vi "Upload File.vi"(7 "Remote Folder Path":string, 8 "error in (no error)":errorcluster, 9 "Connection Name":string, 10 "Local File Path":path, 11 "Remote File Name":string) -> (0 "error out":errorcluster, 3 "Return String":string)   [LabVIEW 2019, in "LabSFTP.lvlib"]
doc: "<License>This software is distributed under the BSD 3-Clause License. For the full license please see license.txt or visit www.labvolution.com/license</License>"
uses:
  LabSFTP.lvlib
  FGV State..enum.ctl
  References/LabSFTP.dll
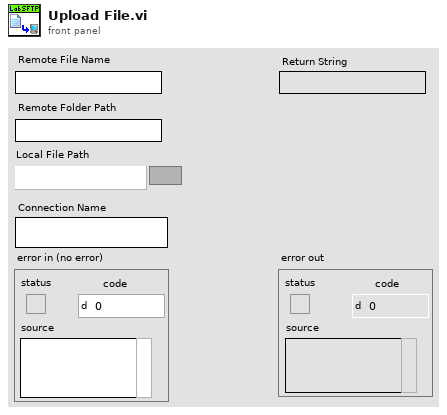
[diagram p1: front panel]
types:
  T1 = typedef "LabSFTP.lvlib/FGV State..enum.ctl" = enum16{"GET", "SET"}
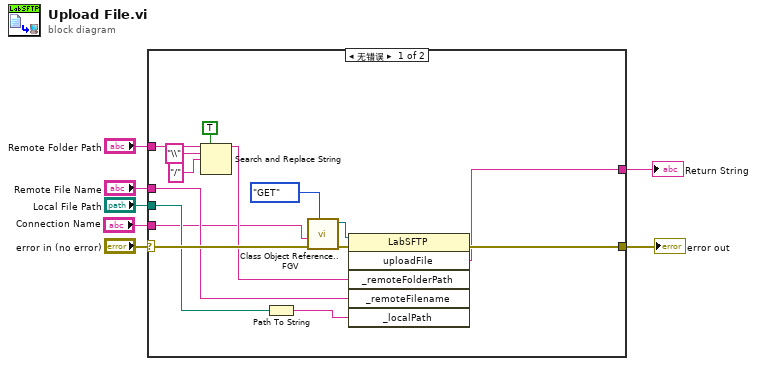
[diagram p0: block diagram]
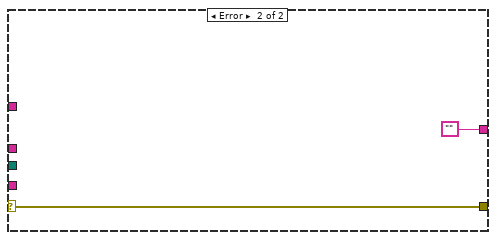
[diagram p2: hidden frame]
diagram:
  n1 = case shown="无错误" "error in (no error)" {
    selector: "error in (no error)" -> [w22 w24]
    tunnel: [w18 w24] -> w6
    tunnel: [w17 ""] -> w5
    tunnel: "Local File Path" -> [w16 _]
    tunnel: "Remote File Name" -> [w15 _]
    tunnel: "Remote Folder Path" -> [w10 _]
    tunnel: "Connection Name" -> [w8 _]
    frame No Error {
      n2 = Search and Replace String(replace all?=TRUE ("replace all? (F)"), input string=w10, search string="\\", replace string="/" ("replace string (\"\")")) -> (result string=w9:string)  [unwired: 4 in, 3 out]
      n3 = Path To String(path=w16) -> (string=w14:string)
      n4 = call "Class Object Reference..FGV.vi"("FGV State"=FGV_State..enum."GET", "error in (no error)"=w22, "Connection Name"=w8) -> ("error out"=w19:errorcluster, "LabSFTP ref out"=w20:refnum<k24>)  [unwired: 7 in]
      n5 = invoke class="LabSFTP" method="uploadFile"(reference=w20, error in=w19, "_remoteFolderPath"=w9, "_remoteFilename"=w15, "_localPath"=w14) -> (error out=w18:errorcluster, "uploadFile"=w17:string)  [unwired: 1 in, 4 out]
    }
    frame Error {
    }
  }
  "error out" <- w6
  "Return String" <- w5
